vi "Read Wavelengths.vi"(8 "error in (no error)":errorcluster, 11 "Spectrometer Driver in":refnum<class "Spectrometer Driver.lvclass">) -> (0 "error out":errorcluster, 2 "Wavelengths":dbl[](array[numeric]), 3 "Spectrometer Driver out":refnum<class "Spectrometer Driver.lvclass">)   [LabVIEW 2016, in "Spectrometer Driver.lvclass"]
uses:
  Spectrometer Driver.lvclass
  Spectrometer Driver.lvclass/Spectrometer Driver.ctl
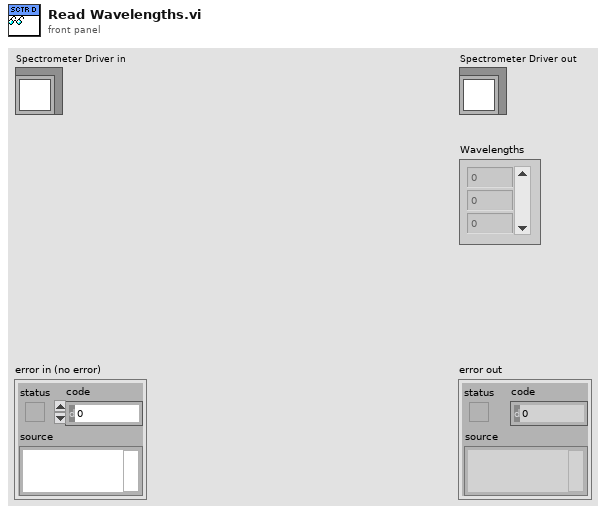
[diagram p1: front panel]
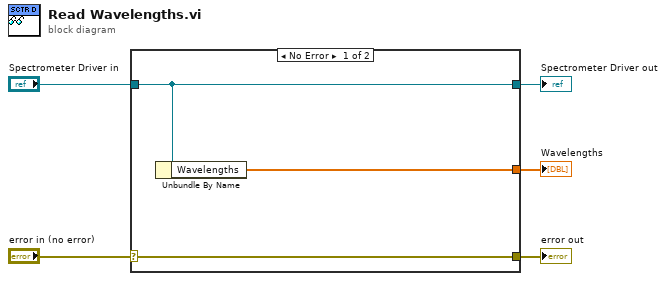
[diagram p0: block diagram]
diagram:
  n1 = case shown="No Error" "error in (no error)" {
    selector: "error in (no error)" -> [w8 w9]
    tunnel: [w8 w9] -> w4
    tunnel: [w7 w10] -> w2
    tunnel: "Spectrometer Driver in" -> [w7 w10]
    tunnel: [w6 _] -> w1
    frame No Error {
      n2 = Unbundle By Name(w7) -> ("Wavelengths"=w6:dbl[])
    }
    frame Error {
    }
  }
  "error out" <- w4
  "Spectrometer Driver out" <- w2
  "Wavelengths" <- w1
